vi "output select rate t str.vi"(11 "rate":u32(ring) items=["APDM_OUTPUT_SELECT_RATE_20", "APDM_OUTPUT_SELECT_RATE_32", "APDM_OUTPUT_SELECT_RATE_40", "APDM_OUTPUT_SELECT_RATE_64", "APDM_OUTPUT_SELECT_RATE_80", "APDM_OUTPUT_SELECT_RATE_128", "APDM_OUTPUT_SELECT_RATE_256", "APDM_OUTPUT_SELECT_RATE_512", "APDM_OUTPUT_SELECT_RATE_640", "APDM_OUTPUT_SELECT_RATE_1280"]) -> (3 "function return":string)   [LabVIEW 2019, in "apdm.lvlib"]
doc: "APDM_EXPORT const char* apdm_output_select_rate_t_str(const apdm_monitor_output_select_rate_t rate);"
uses:
  apdm.lvlib
  Lee Lab/CP FES Walking 2018/Code/Working/LabVIEW/apdm.dll
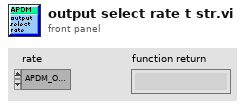
[diagram p1: front panel]
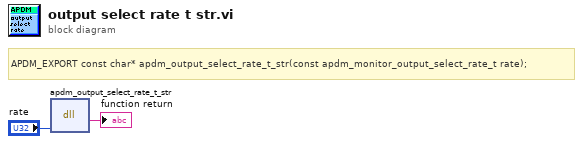
[diagram p0: block diagram]
diagram:
  # "APDM_EXPORT const char* apdm_output_select_rate_t_str(const apdm_monitor_output_select_rate_t rate);"
  n1 = dll-call lib="C:/Users/jfalesi/Dropbox/Lee Lab/CP FES Walking 2018/Code/Working/LabVIEW/apdm.*" fn="apdm_output_select_rate_t_str"("rate"="rate") -> (→"function return":string)  [unwired: 4 in, 2 out]
